vi "PLC String To LV String.vi"(9 "StringLength In PLC":i32=50, 10 "Full String In PLC byte array":u8[](array[numeric]), 11 "Full String In PLC":string) -> (3 "Normal String IN LV":string)   [LabVIEW 2020]
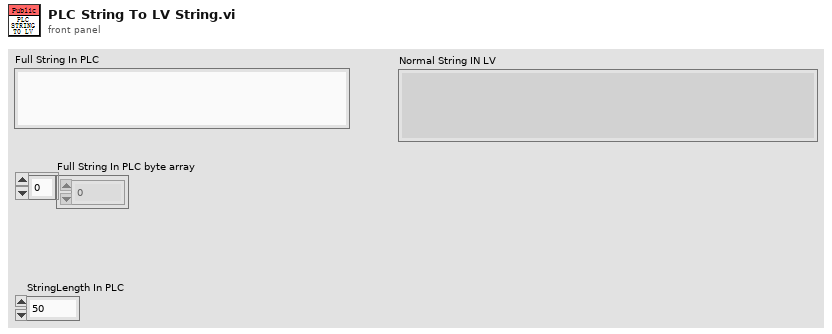
[diagram p1: front panel]
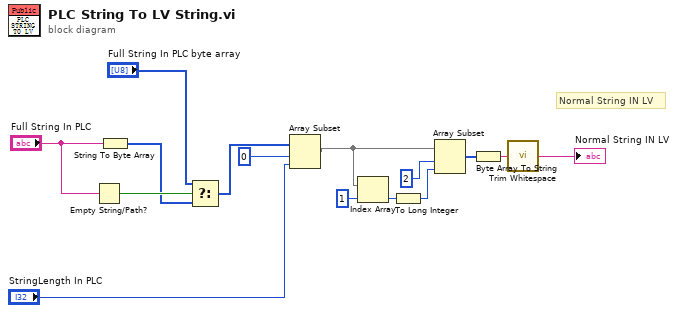
[diagram p0: block diagram]
diagram:
  # "Normal String IN LV"
  n1 = Empty String/Path?(string/path="Full String In PLC") -> (empty?=w4:bool)
  n2 = String To Byte Array(string="Full String In PLC") -> (unsigned byte array=w2:u8[])
  n3 = Select(t="Full String In PLC byte array", s=w4, f=w2) -> (s? t:f=w1:u8[])
  n4 = Array Subset(array=w1, index=0, length="StringLength In PLC") -> (w8:u8[])
  n5 = Index Array(array=w8, index=1) -> (element=w13:u8)
  n6 = To Long Integer(number=w13) -> (32bit integer=w14:i32)
  n7 = Array Subset(array=w8, index=2, length=w14) -> (w10:u8[])
  n8 = Byte Array To String(unsigned byte array=w10) -> (string=w9:string)
  n9 = call <vilib>:"Trim Whitespace.vi"("string"=w9) -> ("trimmed string"=→"Normal String IN LV":string)  [unwired: 1 in]
